vi "Create New Rendezvous.vi"(4 "error in (no error)":errorcluster, 6 "size (2)":i32=2, 7 "name (unnamed)":string) -> (0 "error out":errorcluster, 1 "created new":bool, 3 "rendezvous":T1)   [LabVIEW 2010]
doc: "Looks up an existing rendezvous or creates a new rendezvous and returns a refnum."
uses:
  RendezvousDataCluster.ctl
panel:
  in  "Error Message":string="Create New Rendezvous was asked to create a named Rendezvous already existed."
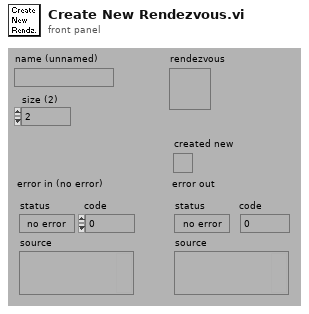
[diagram p1: front panel]
types:
  T1 = typedef "Rendezvous RefNum" = refnum<k1>
  T2 = typedef "RendezvousDataCluster.ctl" = cluster{"Threshold":i32, "Messenger Queues":refnum<queue>[]}
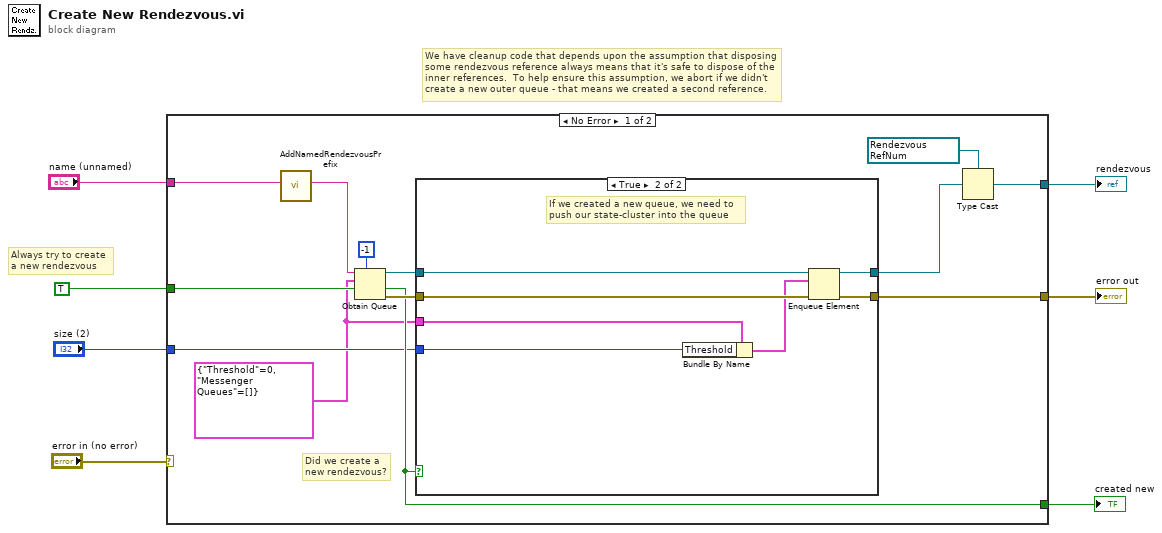
[diagram p0: block diagram]
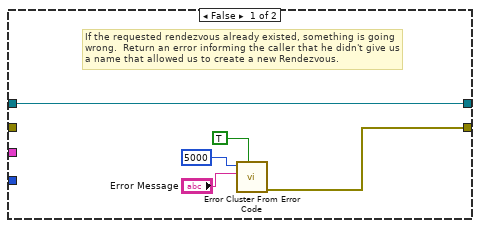
[diagram p2: hidden frame]
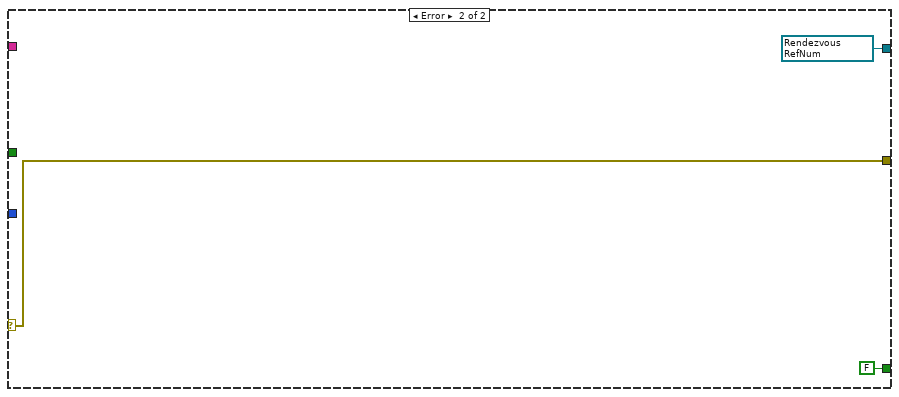
[diagram p3: hidden frame]
diagram:
  # "We have cleanup code that depends upon the assumption that disposing some rendezvous reference always means that it's safe to dispose of the inner references.  To help ensure this assumption, we abort if we didn't create a new outer queue - that means we created a second reference."
  # "Always try to create \na new rendezvous"
  n1 = case shown="No Error" "error in (no error)" {
    selector: "error in (no error)" -> [_ w34]
    tunnel: TRUE -> [w18 _]
    tunnel: "name (unnamed)" -> [w9 _]
    tunnel: [w16 w34] -> w4
    tunnel: [w15 FALSE ("created new?")] -> w5
    tunnel: [w11 w33] -> w6
    tunnel: "size (2)" -> [w14 _]
    frame No Error {
      w13 = T2 {"Threshold"=0, "Messenger Queues"=[]} ("Rendezvous Data-\nClusterTemplate")
      w12 = T1 refnum items=["rendezvous"] ("rendezvous")
      # "Did we create a\nnew rendezvous?"
      n2 = call "AddNamedRendezvousPrefix.vi"("String In"=w9) -> ("String Out"=w8:string)  [unwired: 10 out]
      n3 = Obtain Queue(max queue size (-1, unlimited)=-1, name (unnamed)=w8, element data type=w13, create if not found? (T)=w18) -> (queue out=w20:refnum<queue>, created new?=w15:bool, error out=w19:errorcluster)  [unwired: 1 in]
      n4 = case shown="True" w15 {
        tunnel: w20 -> [w25 w30]
        tunnel: w19 -> [_ w31]
        tunnel: [w25 w29] -> w17
        tunnel: [w24 w28] -> w16
        tunnel: w14 -> [_ w32]
        tunnel: w13 -> [_ w26]
        frame False {
          # "If the requested rendezvous already existed, something is going wrong.  Return an error informing the caller that he didn't give us a name that allowed us to create a new Rendezvous."
          n5 = call "Error Cluster From Error Code.vi"("show call chain? (False)"=TRUE, "error message (\"\")"="Error Message", "error code (0)"=5000) -> ("error out"=w24:errorcluster)  [unwired: 1 in, 5 out]
        }
        frame True {
          # "If we created a new queue, we need to push our state-cluster into the queue"
          n6 = Bundle By Name(cluster=w26, "Threshold"=w32) -> (w27:T2)
          n7 = Enqueue Element(queue=w30, element=w27, error in (no error)=w31) -> (queue out=w29:refnum<queue>, error out=w28:errorcluster)  [unwired: 2 out]
        }
      }
      n8 = Type Cast(type=w12, x=w17) -> (*(type *) &x=w11:T1)
    }
    frame Error {
      w33 = T1 refnum items=["rendezvous"] ("rendezvous")
    }
  }
  "error out" <- w4
  "rendezvous" <- w6
  "created new" <- w5
